vi "Read Parameter File.vi"(8 "error in (no error)":errorcluster, 11 "CD Parameter Manager in":refnum<class "CD Parameter Manager.lvclass">) -> (0 "error out":errorcluster, 3 "CD Parameter Manager out":refnum<class "CD Parameter Manager.lvclass">)   [LabVIEW 2019, in "CD Parameter Manager API.lvlib" / "CD Parameter Manager.lvclass"]
uses:
  CD Parameter Manager.lvclass
  CD Parameter Manager.lvclass/CD Parameter Manager.ctl
  Parameter Generic File/Parameter Generic File.lvclass
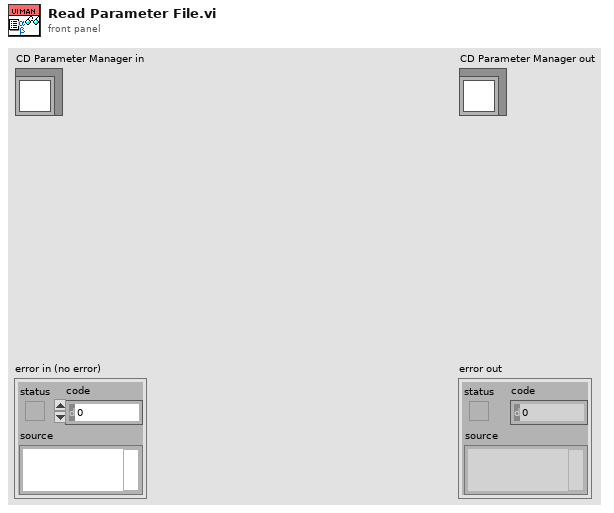
[diagram p1: front panel]
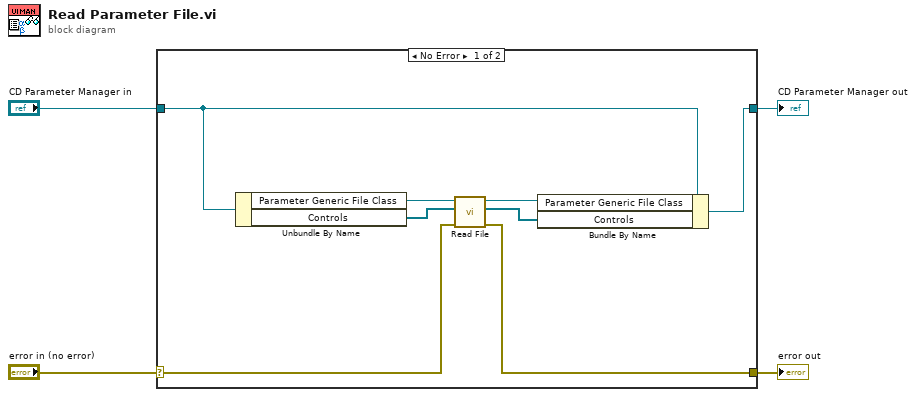
[diagram p0: block diagram]
diagram:
  n1 = case shown="No Error" "error in (no error)" {
    selector: "error in (no error)" -> [w11 w14]
    tunnel: [w10 w14] -> w3
    tunnel: [w7 w13] -> w1
    tunnel: "CD Parameter Manager in" -> [w8 w13]
    frame No Error {
      n2 = Unbundle By Name(w8) -> ("Parameter Generic File Class"=w12:refnum<class "Parameter Generic File.lvclass">, "Controls"=w9:refnum<class "Parameter.lvclass">[])
      n3 = call-dynamic "Read File.vi"("error in (no error)"=w11, "Parameters in"=w9, "Parameter Generic File in"=w12) -> ("error out"=w10:errorcluster, "Parameters out"=w5:refnum<class "Parameter.lvclass">[], "Parameter Generic File out"=w6:refnum<class "Parameter Generic File.lvclass">)  [unwired: 6 in]
      n4 = Bundle By Name(cluster=w8, "Parameter Generic File Class"=w6, "Controls"=w5) -> (w7:refnum<class "CD Parameter Manager.lvclass">)
    }
    frame Error {
    }
  }
  "error out" <- w3
  "CD Parameter Manager out" <- w1
